vi "Send Add Available Measurement.vi"(7 "Message Priority (Normal)":T1=enum."Normal", 8 "error in (no error)":errorcluster, 10 "Name":string, 11 "Message Enqueuer":refnum<class "Message Enqueuer.lvclass">) -> (0 "error out":errorcluster, 3 "Message Enqueuer out":refnum<class "Message Enqueuer.lvclass">)   [LabVIEW 2015, in "Add Available Measurement Msg.lvclass"]
doc: "This VI sends the message to an actor."
uses:
  Add Available Measurement Msg.lvclass
  <vilib>/ActorFramework/Message Enqueuer/Message Enqueuer.lvclass
  <vilib>/ActorFramework/Message Enqueuer/Message Priority.ctl
  Add Available Measurement Msg.lvclass/Add Available Measurement Msg.ctl
  <vilib>/ActorFramework/Message Enqueuer/Message Enqueuer.lvclass/Message Enqueuer.ctl
  <vilib>/ActorFramework/Message Priority Queue/Priority Enqueue.vi
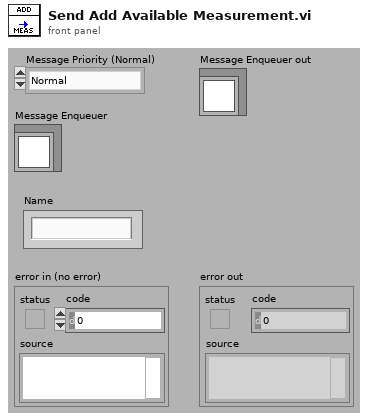
[diagram p1: front panel]
types:
  T1 = typedef "Actor Framework.lvlib/Message Enqueuer.lvclass/Message Priority.ctl" = enum16{"Low", "Normal", "High"}
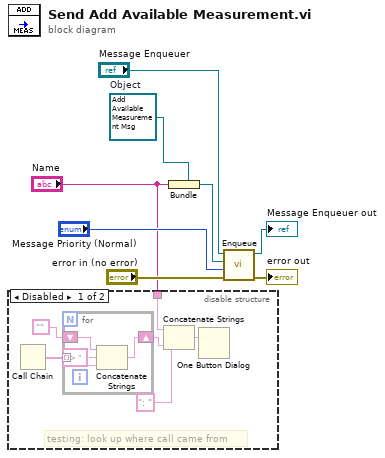
[diagram p0: block diagram]
diagram:
  w5 = refnum<class "Add Available Measurement Msg.lvclass"> refnum  # Object
  n1 = disable-structure shown="Disabled" {
    disable-tunnel: "Name" -> [w11 _]
    frame Disabled {
      # "testing: look up where call came from"
      n2 = Call Chain() -> (call chain=w14:string[])
      n3 = for {
        tunnel: w14 -> [w17] mode=indexing
        shift-right: [w16] -> w10
        shift-left: "" -> [w18]
        n4 = Concatenate Strings(w18, " > " ("string"), w17) -> (w16:string)
      }
      n5 = Concatenate Strings(w11, ": " ("string"), w10) -> (w12:string)
      n6 = One Button Dialog(message=w12) -> ()  [unwired: 1 in, 1 out]
    }
    frame Enabled {
    }
  }
  n7 = Bundle(cluster=w5, "Name") -> (w4:refnum<class "Add Available Measurement Msg.lvclass">)
  n8 = call <vilib>:"Enqueue.vi"("error in (no error)"="error in (no error)", "Message Priority (Normal)"="Message Priority (Normal)", "Message"=w4, "Message Enqueuer in"="Message Enqueuer") -> ("error out"=→"error out":errorcluster, "Message Enqueuer out"=→"Message Enqueuer out":refnum<class "Message Enqueuer.lvclass">)  [unwired: 6 in]
